vi "Destroy.vi"   [LabVIEW 2018, in "Toolkit.lvlib" / "Listener.lvclass"]
doc: "Destroys this Listener object and frees the memory allocated for the libssh2lv shared library Listener struct. No other VIs in the Listener class should be executed once this VI has completed."
uses:
  Listener.lvclass
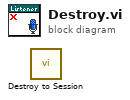
[diagram p0: block diagram]
diagram:
  n1 = call "Destroy to Session.vi"() -> ()  [unwired: 10 in, 2 out]
